vi "Configure Trace Math.vi"(0 "VISA resource name":refnum<visa-resource-name>, 1 "Math Function (0: Off)":i32(ring) items=["Off", "Add", "Subtract"], 5 "Destination Trace (3: Trace 3)":i32(ring)=3 items=["Trace 1"=1, "Trace 2"=2, "Trace 3"=3, "Trace 4"=4], 7 "Source Trace 1 (1: Trace 1)":i32(ring)=1 items=["Trace 1"=1, "Trace 2"=2, "Trace 3"=3, "Trace 4"=4], 9 "Source Trace 2 (2: Trace 2)":i32(ring)=2 items=["Trace 1"=1, "Trace 2"=2, "Trace 3"=3, "Trace 4"=4], 11 "error in (no error)":errorcluster, 12 "Math Type (0: Log Power)":i32(ring) items=["Log Power", "Power"]) -> (4 "VISA resource name out":refnum<visa-resource-name>, 15 "error out":errorcluster)   [LabVIEW 2022 SP3, in "Agilent N934X Series.lvlib"]
doc: "Configure the trace math functions of the spectrum."
uses:
  <instrlib>/Agilent N934X Series/Agilent N934X Series.lvlib
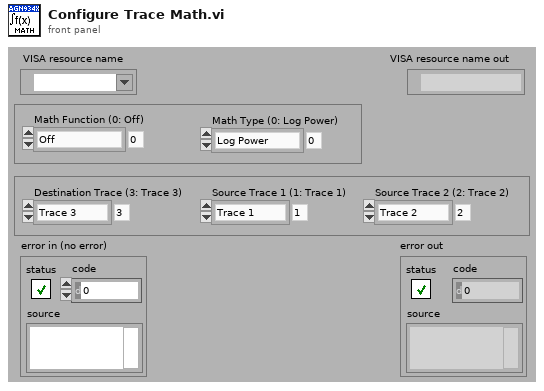
[diagram p1: front panel]
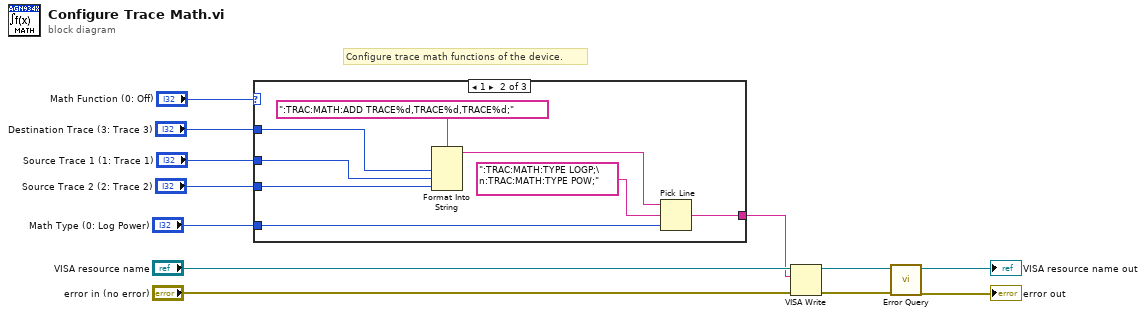
[diagram p0: block diagram]
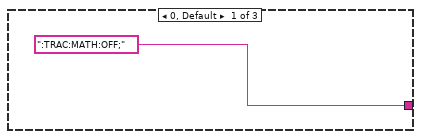
[diagram p2: hidden frame]
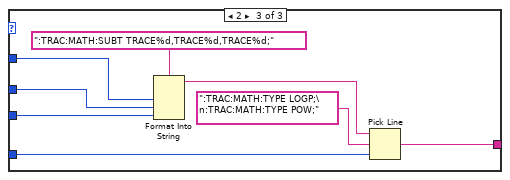
[diagram p3: hidden frame]
diagram:
  # "Configure trace math functions of the device."
  n1 = case shown="1" "Math Function (0: Off)" {
    tunnel: "Destination Trace (3: Trace 3)" -> [_ w21 w29]
    tunnel: "Source Trace 1 (1: Trace 1)" -> [_ w20 w28]
    tunnel: "Source Trace 2 (2: Trace 2)" -> [_ w19 w24]
    tunnel: "Math Type (0: Log Power)" -> [_ w16 w23]
    tunnel: [":TRAC:MATH:OFF;" w15 w22] -> w1
    frame 0, Default {
    }
    frame 1 {
      n2 = Format Into String(format string=":TRAC:MATH:ADD TRACE%d,TRACE%d,TRACE%d;", w21, w20, w19) -> (resulting string=w18:string)  [unwired: 2 in, 1 out]
      n3 = Pick Line(string ("")=w18, multi-line string=":TRAC:MATH:TYPE LOGP;\n:TRAC:MATH:TYPE POW;", line index=w16) -> (output string=w15:string)
    }
    frame 2 {
      n4 = Format Into String(format string=":TRAC:MATH:SUBT TRACE%d,TRACE%d,TRACE%d;", w29, w28, w24) -> (resulting string=w26:string)  [unwired: 2 in, 1 out]
      n5 = Pick Line(string ("")=w26, multi-line string=":TRAC:MATH:TYPE LOGP;\n:TRAC:MATH:TYPE POW;", line index=w23) -> (output string=w22:string)
    }
  }
  n6 = VISA Write(VISA resource name="VISA resource name", write buffer=w1, error in (no error)="error in (no error)") -> (VISA resource name out=w10:refnum<visa-resource-name>, error out=w9:errorcluster)  [unwired: 1 out]
  n7 = call <instrlib>:"Error Query.vi"("error in (no error)"=w9, "VISA resource name"=w10) -> ("error out"=→"error out":errorcluster, "VISA resource name out"=→"VISA resource name out":refnum<visa-resource-name>)  [unwired: 6 in, 2 out]
